vi "Exercises_4-1.vi"() -> ()   [LabVIEW 2014]
panel:
  out "Warning?":bool
  out "Warning Text":string
  in  "Min Temp":dbl
  in  "Max Temp":dbl
  in  "Current Temp":dbl
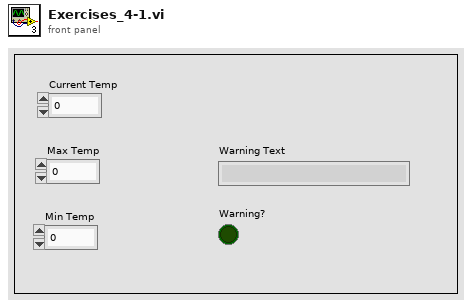
[diagram p1: front panel]
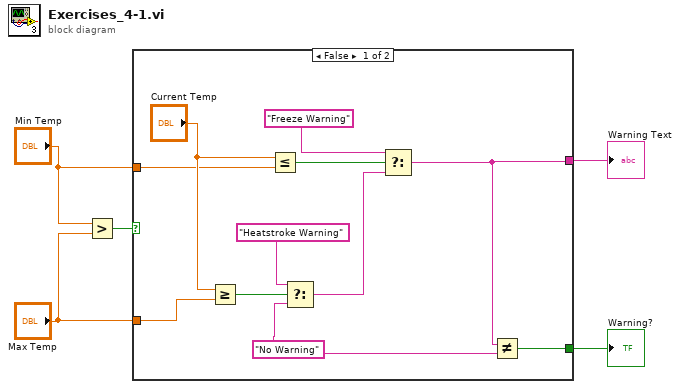
[diagram p0: block diagram]
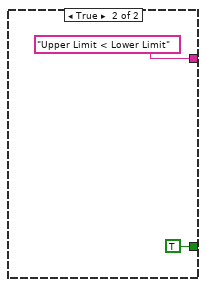
[diagram p2: hidden frame]
diagram:
  n1 = Greater?(x="Min Temp", y="Max Temp") -> (0:w1:bool)
  n2 = case shown="False" w1 {
    tunnel: [w10 "Upper Limit < Lower Limit"] -> w5
    tunnel: [w8 TRUE] -> w4
    tunnel: "Min Temp" -> [w7 _]
    tunnel: "Max Temp" -> [w6 _]
    frame False {
      w9 = "No Warning"
      n3 = Greater Or Equal?(x="Current Temp", y=w6) -> (x >= y?=w16:bool)
      n4 = Less Or Equal?(x="Current Temp", y=w7) -> (x <= y?=w13:bool)
      n5 = Select(t="Heatstroke Warning", s=w16, f=w9) -> (s? t:f=w12:string)
      n6 = Select(t="Freeze Warning", s=w13, f=w12) -> (s? t:f=w10:string)
      n7 = Not Equal?(x=w10, y=w9) -> (x != y?=w8:bool)
    }
    frame True {
    }
  }
  "Warning Text" <- w5
  "Warning?" <- w4
